vi "DB Import Action - Create Chans.vi"(8 "error in (no error)":errorcluster, 10 "selected path":path, 11 "Node Ptr":u64) -> (0 "error out":errorcluster, 2 "selected path out":path caption="selected path", 3 "Node Ptr dup":u64)   [LabVIEW 2015, in "AIT 429 System Explorer.lvlib"]
uses:
  AIT 429 System Explorer.lvlib
  Create Sysdef Tree Labels.vi
  Build Label Properties.vi
  AddParamChannels.vi
  <vilib>/NI Veristand/Custom Device API/NI VeriStand - Add Custom Device Section.vi
  <vilib>/NI Veristand/Custom Device API/NI VeriStand - Add Custom Device Channel.vi
  Shared/Controls and Global/Global.vi
  <vilib>/NI Veristand/Custom Device Tools/Custom Device Utility Library/NI VeriStand - Search for Item.vi
  <vilib>/NI Veristand/Custom Device Tools/Custom Device Utility Library/NI VeriStand - Search for Item by GUID.vi
  <vilib>/NI Veristand/Custom Device API/Custom Device API.lvlib
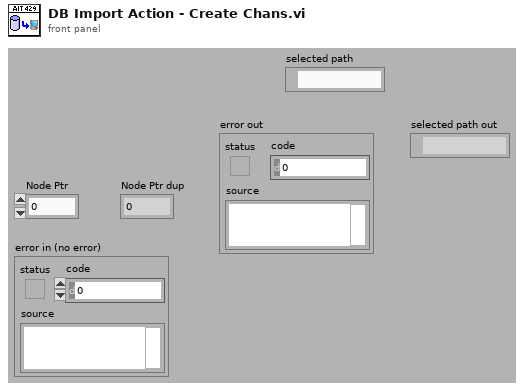
[diagram p1: front panel]
types:
  T1 = typedef "AIT 429 System Explorer.lvlib/AIT_Channel Array.ctl" = T2[]
  T2 = typedef "AIT 429 System Explorer.lvlib/AIT_Channel.ctl" = cluster{"Labels":T3[], "name":string, "number":u8, "direction":enum16{"OWL429_DIRECTION_RX", "OWL429_DIRECTION_TX"}, "Voltage":dbl, "speed":T7}
  T3 = typedef "AIT 429 System Explorer.lvlib/AIT_Label.ctl" = cluster{"name":string, "xmlName":string, "TxPeriod":u32, "label":u32, "TxRate":dbl, "SDI_Enabled":bool, "SDIValue":u8, "BufferSize":u32, "Words":T4[], "TransferType":T6}
  T4 = typedef "AIT 429 System Explorer.lvlib/AIT_Word.ctl" = cluster{"InitalValue":u32, "Params":T5[]}
  T5 = typedef "AIT 429 System Explorer.lvlib/ARINCParam.ctl" = cluster{"name":string, "startBit":i32, "numberBits":i32, "scaleFactor":dbl, "scaleOffset":dbl, "signed":bool}
  T6 = typedef "AIT 429 Shared.lvlib/TransferType.ctl" = enum16{"ScheduledLabel", "Acyclic", "Block", "Strobe"}
  T7 = typedef "Owl429.lvlib/Owl429ChannelSpeed.ctl" = enum16{"OWL429_HIGH_SPEED_CHANNEL", "OWL429_LOW_SPEED_CHANNEL"}
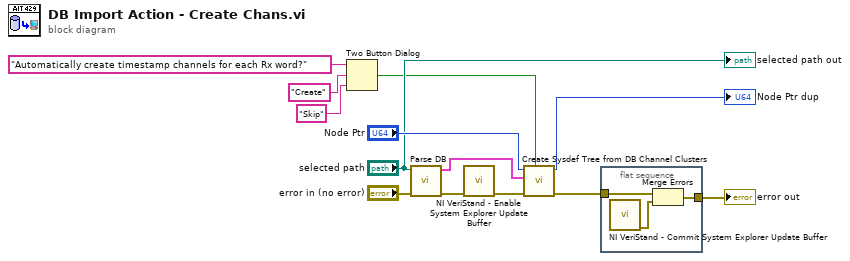
[diagram p0: block diagram]
diagram:
  n1 = Two Button Dialog(message="Automatically create timestamp channels for each Rx word?", 1:"Skip" ("F button name (\"Cancel\")"), 2:"Create" ("T button name (\"OK\")")) -> (T button?=w1:bool)
  n2 = call "Parse DB.vi"("error in (no error)"="error in (no error)", "Path in"="selected path") -> ("error out"=w8:errorcluster, "channels"=w12:T1)  [unwired: 8 in]
  n3 = call <vilib>:"NI VeriStand - Enable System Explorer Update Buffer.vi"("error in (no error)"=w8) -> ("error out"=w11:errorcluster)  [unwired: 10 in]
  n4 = call "Create Sysdef Tree from DB Channel Clusters.vi"("Autocreate Rx timestamp chans?"=w1, "error in"=w11, "Channels to create"=w12, "Device Ptr"="Node Ptr") -> ("error out"=w6:errorcluster, "Device Ptr dup"=→"Node Ptr dup":u64)  [unwired: 6 in]
  n5 = flat-sequence {
    tunnel: w6 -> [w16]
    tunnel: [w14] -> w5
    frame #0 {
      n6 = call <vilib>:"NI VeriStand - Commit System Explorer Update Buffer.vi"() -> ("error out"=w15:errorcluster)  [unwired: 11 in]
      n7 = Merge Errors(w16, w15) -> (w14:errorcluster)
    }
  }
  "error out" <- w5
  "selected path out" <- "selected path"
